vi "poly_signalling_write_single.vi"(6 "mode (Sgnl)":T1(ring)=enum."Val(Sgnl)", 8 "error in (no error)":errorcluster, 9 "Value":variant, 10 "Control Name":string, 11 "vi reference":refnum<vi>) -> (0 "error out":errorcluster, 2 "controll reference out":refnum<vi>, 3 "vi reference out":refnum<vi>, 4 "found?":bool)   [LabVIEW 2015]
uses:
  poly_control_ref_from_name_single.vi
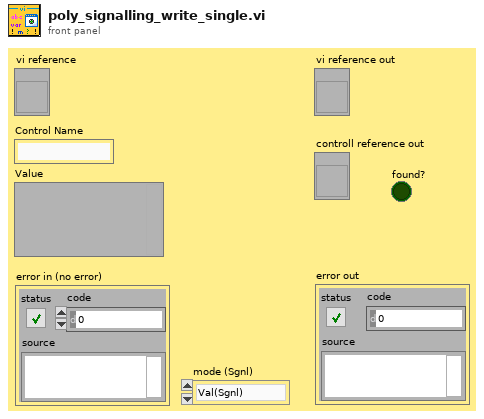
[diagram p1: front panel]
types:
  T1 = enum16{"Val", "Val(Sgnl)", "Val(Undo)", "Method"}
  T2 = enum16{"Val", "Val(Sgnl)", "Val(Undo)", "Method"}[]
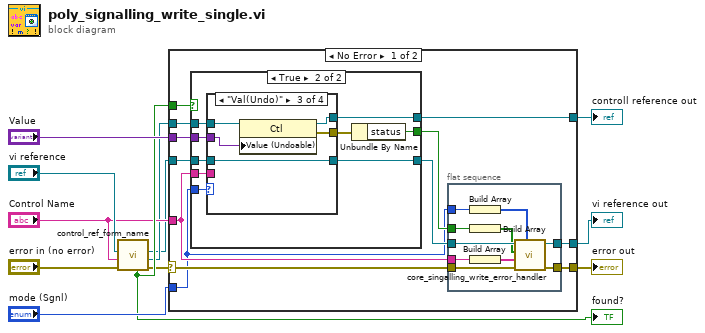
[diagram p0: block diagram]
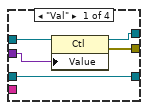
[diagram p3: hidden frame]
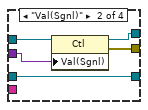
[diagram p4: hidden frame]
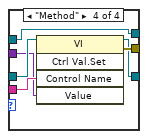
[diagram p5: hidden frame]
diagram:
  n1 = call-poly "control_ref_form_name.vi"("error in (no error)"="error in (no error)", "control name"="Control Name", "vi ref"="vi reference") -> ("error out"=w1:errorcluster, "ctrl ref"=w3:refnum<vi>, "vi ref dup"=w2:refnum<vi>, "found?"=w7:bool)  [unwired: 5 in]
  "found?" <- w7
  n2 = case shown="No Error" w1 {
    selector: w1 -> [w19 w70]
    tunnel: "Value" -> [w24 _]
    tunnel: "mode (Sgnl)" -> [w13 _]
    tunnel: [w18 w70] -> w10
    tunnel: [w23 w68] -> w9
    tunnel: [w16 w69] -> w8
    tunnel: w7 -> [w22 _]
    tunnel: "Control Name" -> [w14 _]
    tunnel: w3 -> [w21 w68]
    tunnel: w2 -> [w20 w69]
    frame No Error {
      n3 = case shown="True" w22 {
        selector: w22 -> [w35 _]
        tunnel: w24 -> [_ w46]
        tunnel: w13 -> [_ w45]
        tunnel: [w35 w38] -> w15
        tunnel: [w36 w44] -> w23
        tunnel: [w37 w43] -> w17
        tunnel: w14 -> [_ w42]
        tunnel: w20 -> [w37 w41]
        tunnel: w21 -> [w36 w40]
        frame False {
        }
        frame True {
          n4 = case shown="\"Val(Undo)\"" w45 {
            tunnel: w40 -> [w51 w53 w60 w65]
            tunnel: w46 -> [w50 w56 w61 w62]
            tunnel: [w49 w55 w57 w66] -> w39
            tunnel: [w48 w54 w59 w65] -> w44
            tunnel: w41 -> [w47 w52 w58 w67]
            tunnel: [w47 w52 w58 w64] -> w43
            tunnel: w42 -> [_ _ _ w63]
            frame "Val" {
              n5 = property class="Ctl"(reference=w51, "Value"=w50) -> (reference out=w48:refnum<vi>, error out=w49:errorcluster)  [unwired: 1 in]
            }
            frame "Val(Sgnl)" {
              n6 = property class="Ctl"(reference=w53, "Val(Sgnl)"=w56) -> (reference out=w54:refnum<vi>, error out=w55:errorcluster)  [unwired: 1 in]
            }
            frame "Val(Undo)" {
              n7 = property class="Ctl"(reference=w60, "Value (Undoable)"=w61) -> (reference out=w59:refnum<vi>, error out=w57:errorcluster)  [unwired: 1 in]
            }
            frame "Method" {
              n8 = invoke class="VI" method="Ctrl Val.Set"(reference=w67, "Control Name"=w63, "Value"=w62) -> (reference out=w64:refnum<vi>, error out=w66:errorcluster)  [unwired: 2 in, 3 out]
            }
          }
          n9 = Unbundle By Name(w39) -> ("status"=w38:bool)
        }
      }
      n10 = flat-sequence {
        tunnel: w19 -> [w34]
        tunnel: [w33] -> w18
        tunnel: w17 -> [w32]
        tunnel: [w31] -> w16
        tunnel: w15 -> [w30]
        tunnel: w14 -> [w28]
        tunnel: w13 -> [w26]
        frame #0 {
          n11 = Build Array(w26) -> (w25:T2)
          n12 = Build Array(w30) -> (w29:bool[])
          n13 = Build Array(w28) -> (w27:string[])
          n14 = call "core_singalling_write_error_handler.vi"("modes (Sgnl)"=w25, "error in"=w34, "control names"=w27, "error?"=w29, "vi ref"=w32) -> ("error out"=w33:errorcluster, "vi ref dup"=w31:refnum<vi>)  [unwired: 5 in]
        }
      }
    }
    frame Error {
    }
  }
  "error out" <- w10
  "vi reference out" <- w8
  "controll reference out" <- w9
